vi "APE_tcp client.vi"(7 "Action":T1, 8 "error in":errorcluster, 9 "Command":string, 10 "TCP Port":u16=51019, 11 "Host":string) -> (0 "error out":errorcluster, 1 "Answer":string)   [LabVIEW 2026]
doc: "# #############################################################################\n# ATTENTION\n# #############################################################################\n#\n# This software is for guidance only. It is provided \"as is\".\n# It only aims at providing coding information to the customer in order for\n# them to save time. As a result no warranties, whether express, implied or\n# statutory, including, but not limited to implied warranties of\n# merchantability and fitness for a particular purpose apply to this software.\n# A·P·E Angewandte Physik und Elektronik GmbH shall not be held liable for any\n# direct, indirect or consequential damages with respect to any claims arising\n# from the content of such sourcecode and/or the use made by customers of the\n# coding information contained herein in connection with their products.\n#\n# File Version: 1.0\n#\n# Changelog:\n# 1.0 - Initial Version\n#\n# #############################################################################"
uses:
  APE codes/LabVIEW/LV13/Basic Example/cluster/tcp client action.ctl
  APE codes/LabVIEW/LV13/Basic Example/cluster/tcp client data cluster.ctl
  <vilib>/Utility/error.llb/Trim Whitespace One-Sided.vi
  <vilib>/regexp/Match Regular Expression.xnode
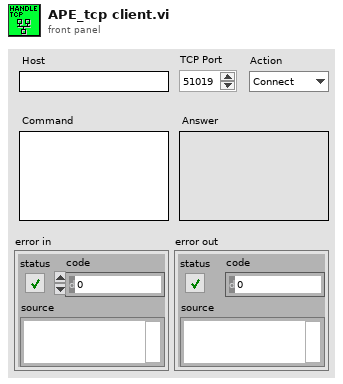
[diagram p1: front panel]
types:
  T1 = typedef "tcp client action.ctl" = enum16{"Connect", "Write", "Query", "Disconnect"}
  T2 = typedef "tcp client data cluster.ctl" = cluster{"connection ID":refnum<k5>, "Host":string, "TCP Port":u16}
  T3 = enum16{"Standard", "Buffered", "CRLF", "Immediate"}
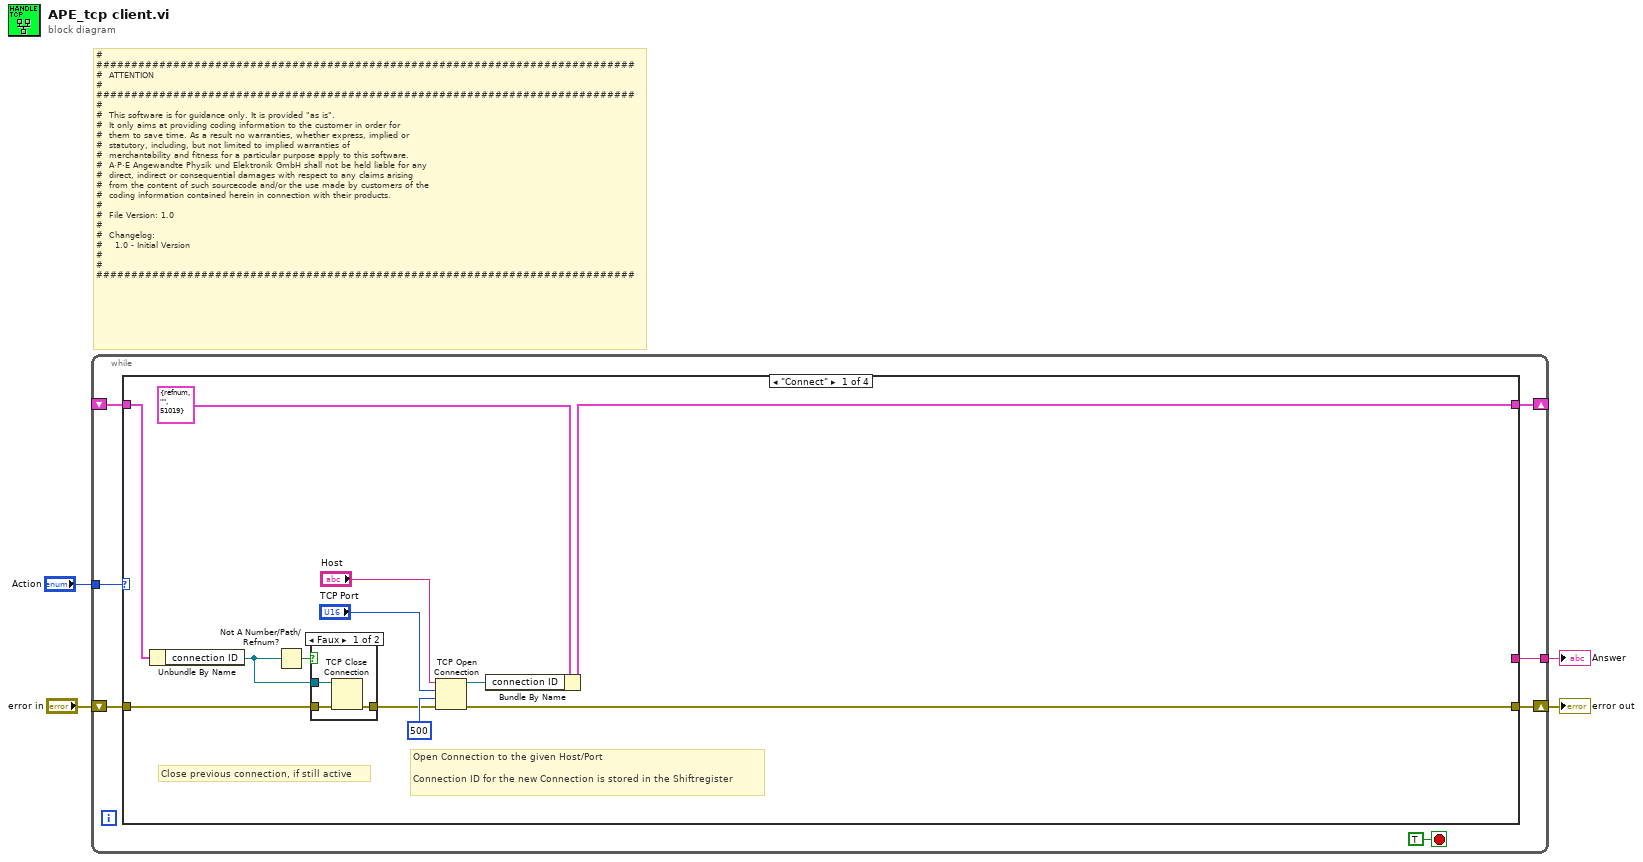
[diagram p0: block diagram]
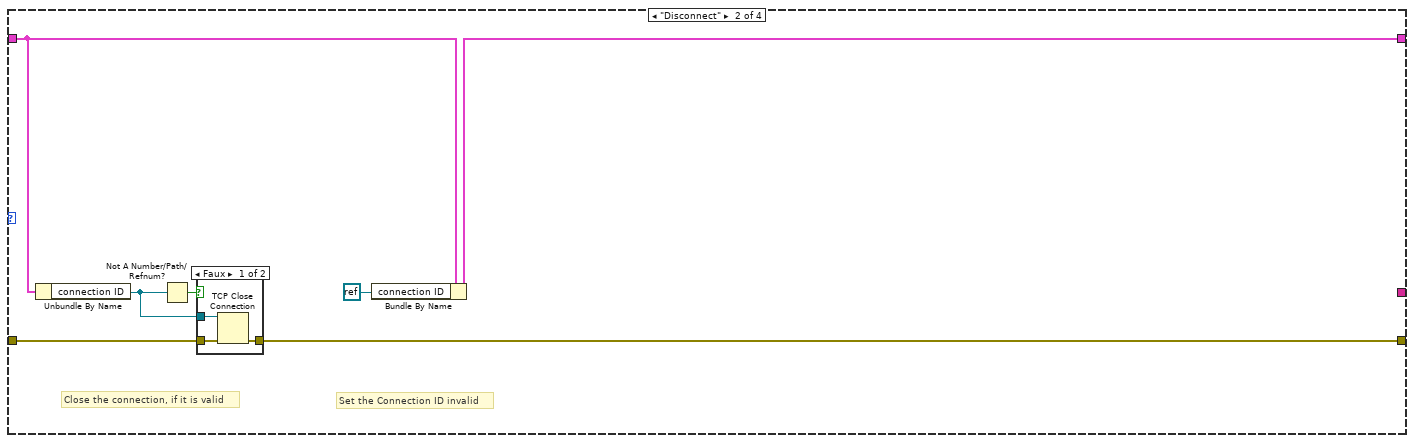
[diagram p3: hidden frame]
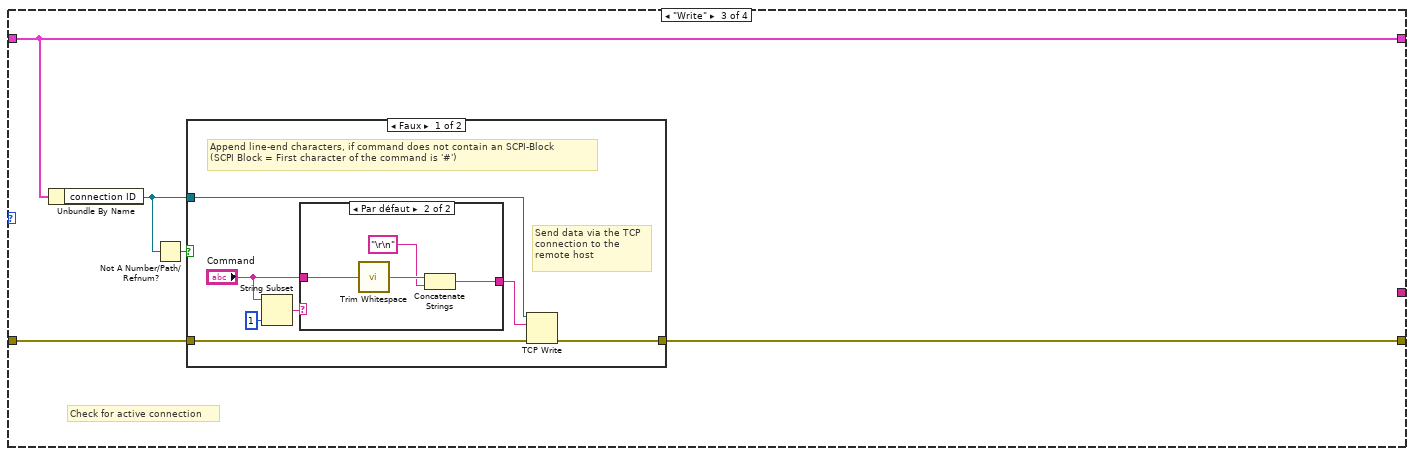
[diagram p5: hidden frame]
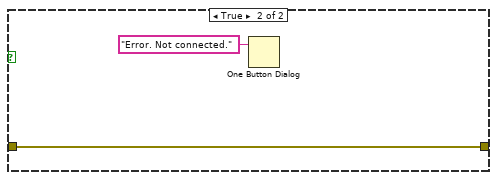
[diagram p7: hidden frame]
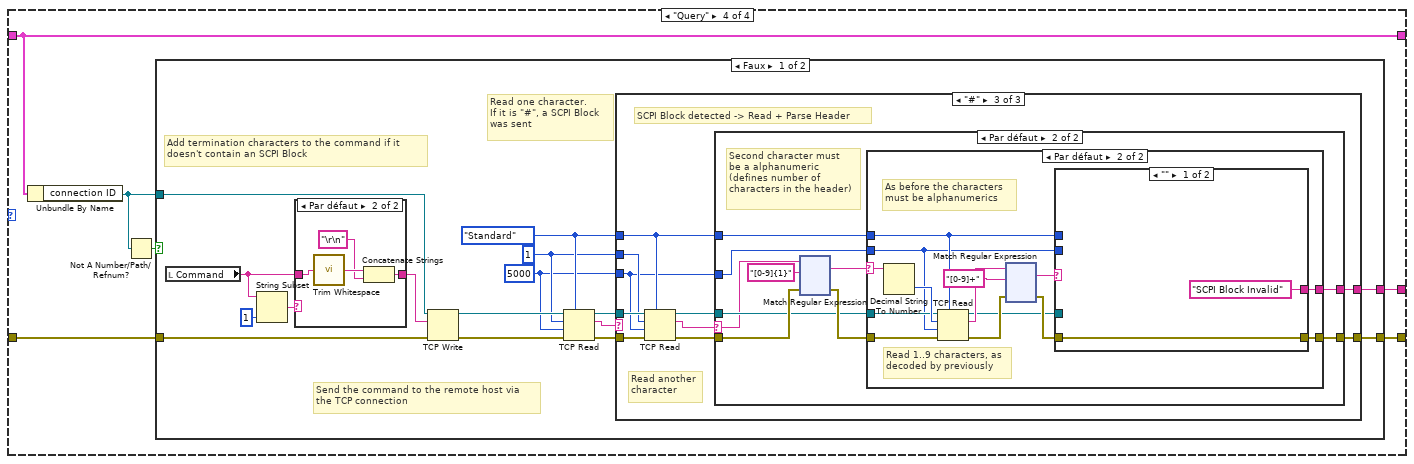
[diagram p8: hidden frame]
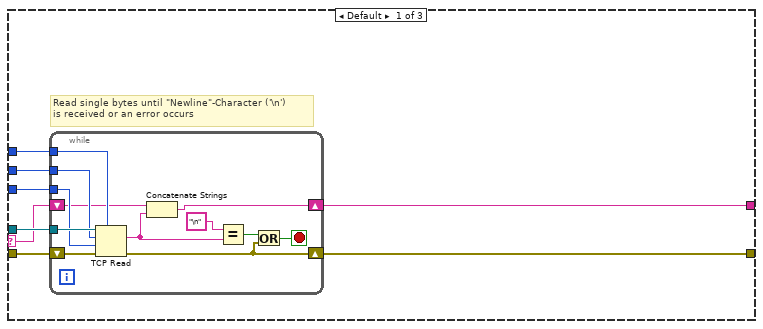
[diagram p9: hidden frame]
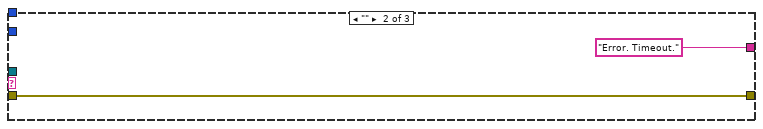
[diagram p10: hidden frame]
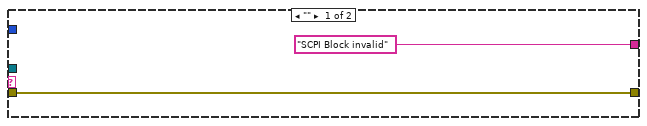
[diagram p11: hidden frame]
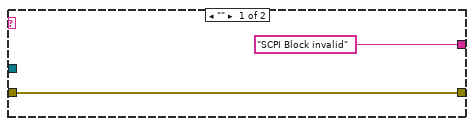
[diagram p12: hidden frame]
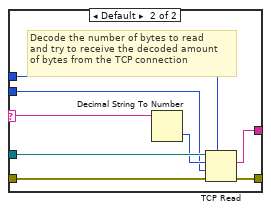
[diagram p13: hidden frame]
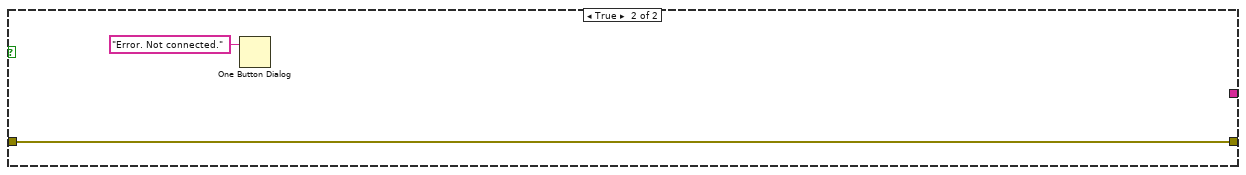
[diagram p15: hidden frame]
diagram:
  # "# #############################################################################\n#  ATTENTION\n# #############################################################################\n#\n#  This software is for guidance only. It is provided \"as is\".\n#  It only aims at providing coding information to the customer in order for\n#  them to save time. As a result no warranties, whether express, implied or\n#  statutory, including, but not limited to implied warranties of\n#  merchantability and fitness for a particular purpose apply to this software.\n#  A·P·E Angewandte Physik und Elektronik GmbH shall not be held liable for any\n#  direct, indirect or consequential damages with respect to any claims arising\n#  from the content of such sourcecode and/or the use made by customers of the\n#  coding information contained herein in connection with their products.\n#\n#  File Version: 1.0\n#\n#  Changelog:\n#    1.0 - Initial Version\n#\n# #############################################################################"
  n1 = while {
    shift-right: [w10] -> _
    shift-left: _ -> [w9]
    shift-right: [w8] -> w3
    shift-left: "error in" -> [w7]
    tunnel: "Action" -> [w6]
    tunnel: [w5] -> w1
    stop <- TRUE stop-if-true
    n2 = case shown="\"Connect\"" w6 {
      tunnel: [w15 w31 w40 w60] -> w10
      tunnel: w9 -> [w16 w28 w40 w60]
      tunnel: [w17 w30 w43 w63] -> w8
      tunnel: w7 -> [w20 w32 w42 w62]
      tunnel: [_ _ _ w58] -> w5
      frame "Connect" {
        # "Open Connection to the given Host/Port\n\nConnection ID for the new Connection is stored in the Shiftregister"
        # "Close previous connection, if still active"
        n3 = Unbundle By Name(w16) -> ("connection ID"=w21:refnum<k5>)
        n4 = Not A Number/Path/Refnum?(number/path/refnum=w21) -> (NaN/Path/Refnum?=w22:bool)
        n5 = case shown="Faux" w22 {
          tunnel: w21 -> [w26 _]
          tunnel: w20 -> [w25 w27]
          tunnel: [w24 w27] -> w18
          frame False {
            n6 = TCP Close Connection(connection ID=w26, error in (no error)=w25) -> (error out=w24:errorcluster)  [unwired: 1 in, 1 out]
          }
          frame True {
          }
        }
        n7 = TCP Open Connection(address="Host", remote port or service name="TCP Port", timeout ms (60000)=500, error in (no error)=w18) -> (connection ID=w14:refnum<k5>, error out=w17:errorcluster)  [unwired: 1 in]
        n8 = Bundle By Name(cluster=T2 {"connection ID"=refnum, "Host"="", "TCP Port"=51019}, "connection ID"=w14) -> (w15:T2)
      }
      frame "Disconnect" {
        # "Set the Connection ID invalid"
        # "Close the connection, if it is valid"
        n9 = Unbundle By Name(w28) -> ("connection ID"=w33:refnum<k5>)
        n10 = Not A Number/Path/Refnum?(number/path/refnum=w33) -> (NaN/Path/Refnum?=w34:bool)
        n11 = case shown="Faux" w34 {
          tunnel: w33 -> [w37 _]
          tunnel: w32 -> [w36 w38]
          tunnel: [w35 w38] -> w30
          frame False {
            n12 = TCP Close Connection(connection ID=w37, error in (no error)=w36) -> (error out=w35:errorcluster)  [unwired: 1 in, 1 out]
          }
          frame True {
          }
        }
        n13 = Bundle By Name(cluster=w28, "connection ID"=refnum<k0> refnum) -> (w31:T2)
      }
      frame "Write" {
        # "Check for active connection"
        n14 = Unbundle By Name(w40) -> ("connection ID"=w39:refnum<k5>)
        n15 = Not A Number/Path/Refnum?(number/path/refnum=w39) -> (NaN/Path/Refnum?=w41:bool)
        n16 = case shown="Faux" w41 {
          tunnel: [w46 w57] -> w43
          tunnel: w42 -> [w47 w57]
          tunnel: w39 -> [w45 _]
          frame False {
            # "Send data via the TCP\nconnection to the \nremote host"
            # "Append line-end characters, if command does not contain an SCPI-Block\n(SCPI Block = First character of the command is '#')"
            n17 = String Subset(string="Command", length (rest)=1 ("length (rest)")) -> (substring=w48:string)  [unwired: 1 in]
            n18 = case shown="Par défaut" w48 {
              tunnel: [w51 w55] -> w50
              tunnel: "Command" -> [w51 w54]
              frame "#" {
              }
              frame Default {
                n19 = call <vilib>:"Trim Whitespace.vi"("string"=w54) -> ("trimmed string"=w53:string)  [unwired: 1 in]
                n20 = Concatenate Strings(w53, "\r\n" ("termination")) -> (w55:string)
              }
            }
            n21 = TCP Write(connection ID=w45, data in=w50, error in (no error)=w47) -> (error out=w46:errorcluster)  [unwired: 1 in, 2 out]
          }
          frame True {
            n22 = One Button Dialog(message="Error. Not connected.") -> ()  [unwired: 1 in, 1 out]
          }
        }
      }
      frame "Query" {
        n23 = Unbundle By Name(w60) -> ("connection ID"=w59:refnum<k5>)
        n24 = Not A Number/Path/Refnum?(number/path/refnum=w59) -> (NaN/Path/Refnum?=w61:bool)
        n25 = case shown="Faux" w61 {
          tunnel: [w70 w390] -> w63
          tunnel: w62 -> [w76 w390]
          tunnel: w59 -> [w75 _]
          tunnel: [w64 _] -> w58
          frame False {
            w65 = 5000 ("timeout ms (25000)")
            w66 = 1 ("bytes to read")
            w67 = T3."Standard" ("mode (standard)")
            # "Send the command to the remote host via\nthe TCP connection"
            # "Add termination characters to the command if it \ndoesn't contain an SCPI Block"
            # "Read one character.\nIf it is \"#\", a SCPI Block \nwas sent"
            n26 = local read "Command"() -> (w74:string)
            n27 = String Subset(string=w74, length (rest)=1 ("length (rest)")) -> (substring=w77:string)  [unwired: 1 in]
            n28 = case shown="Par défaut" w77 {
              tunnel: [w384 w388] -> w79
              tunnel: w74 -> [w384 w387]
              frame "#" {
              }
              frame Default {
                n29 = call <vilib>:"Trim Whitespace.vi"("string"=w387) -> ("trimmed string"=w386:string)  [unwired: 1 in]
                n30 = Concatenate Strings(w386, "\r\n" ("termination")) -> (w388:string)
              }
            }
            n31 = TCP Write(connection ID=w75, data in=w79, error in (no error)=w76) -> (connection ID out=w72:refnum<k5>, error out=w73:errorcluster)  [unwired: 1 in, 1 out]
            n32 = TCP Read(connection ID=w72, bytes to read=w66, error in (no error)=w73, 7:w67, 9:w65) -> (connection ID out=w68:refnum<k5>, data out=w69:string, error out=w71:errorcluster)
            n33 = case shown="\"#\"" w69 {
              selector: w69 -> [w81 _ _]
              tunnel: w71 -> [w87 w100 w111]
              tunnel: [w86 w100 w106] -> w70
              tunnel: w68 -> [w85 _ w110]
              tunnel: w67 -> [w84 _ w103]
              tunnel: w66 -> [w83 _ w109]
              tunnel: w65 -> [w82 _ w102]
              tunnel: [w80 "Error. Timeout." ("data out") w105] -> w64
              frame Default {
                # "Read single bytes until \"Newline\"-Character ('\\n')\nis received or an error occurs"
                n34 = while {
                  tunnel: w85 -> [w98]
                  shift-right: [w88] -> w86
                  shift-left: w87 -> [w99]
                  tunnel: w84 -> [w97]
                  tunnel: w83 -> [w96]
                  tunnel: w82 -> [w95]
                  shift-right: [w93] -> w80
                  shift-left: w81 -> [w94]
                  stop <- w89 stop-if-true
                  n35 = TCP Read(connection ID=w98, bytes to read=w96, error in (no error)=w99, 7:w97, 9:w95) -> (data out=w92:string, error out=w88:errorcluster)  [unwired: 1 out]
                  n36 = Concatenate Strings(w94, w92) -> (w93:string)
                  n37 = Equal?(x="\n" ("y"), y=w92) -> (x = y?=w90:bool)
                  n38 = Or(x=w90, y=w88) -> (x .or. y?=w89:bool)
                }
              }
              frame "" {
              }
              frame "#" {
                # "Read another\ncharacter"
                # "SCPI Block detected -> Read + Parse Header"
                n39 = TCP Read(connection ID=w110, bytes to read=w109, error in (no error)=w111, 7:w103, 9:w102) -> (connection ID out=w104:refnum<k5>, data out=w107:string, error out=w108:errorcluster)
                n40 = case shown="Par défaut" w107 {
                  selector: w107 -> [_ w114]
                  tunnel: w108 -> [w112 w123]
                  tunnel: [w112 w116] -> w106
                  tunnel: ["SCPI Block invalid" w115] -> w105
                  tunnel: w104 -> [_ w120]
                  tunnel: w103 -> [_ w119]
                  tunnel: w102 -> [_ w118]
                  frame "" {
                  }
                  frame Default {
                    # "Second character must \nbe a alphanumeric\n(defines number of \ncharacters in the header)"
                    n41 = xnode "Match Regular Expression"("chaîne en entrée"=w114, "expression régulière"="[0-9]{1}" ("regular expression"), "entrée d'erreur"=w123) -> ("toute l'expression"=w117:string, "sortie d'erreur"=w121:errorcluster)  [unwired: 3 in, 3 out]
                    n42 = case shown="Par défaut" w117 {
                      selector: w117 -> [_ w136]
                      tunnel: w121 -> [w125 w138]
                      tunnel: w120 -> [_ w137]
                      tunnel: w119 -> [_ w128]
                      tunnel: w118 -> [_ w127]
                      tunnel: [w125 w131] -> w116
                      tunnel: ["SCPI Block invalid" ("data out") w126] -> w115
                      frame "" {
                      }
                      frame Default {
                        # "As before the characters \nmust be alphanumerics"
                        # "Read 1..9 characters, as \ndecoded by previously"
                        n43 = Decimal String To Number(string=w136) -> (number=w139:i32)  [unwired: 2 in, 1 out]
                        n44 = TCP Read(connection ID=w137, bytes to read=w139, error in (no error)=w138, 7:w128, 9:w127) -> (connection ID out=w129:refnum<k5>, data out=w133:string, error out=w134:errorcluster)
                        n45 = xnode "Match Regular Expression"("chaîne en entrée"=w133, "expression régulière"="[0-9]+" ("regular expression"), "entrée d'erreur"=w134) -> ("toute l'expression"=w130:string, "sortie d'erreur"=w132:errorcluster)  [unwired: 3 in, 3 out]
                        n46 = case shown="\"\"" w130 {
                          selector: w130 -> [_ w146]
                          tunnel: w132 -> [w140 w149]
                          tunnel: [w140 w148] -> w131
                          tunnel: w129 -> [_ w147]
                          tunnel: w128 -> [_ w145]
                          tunnel: w127 -> [_ w143]
                          tunnel: ["SCPI Block Invalid" ("data out") w142] -> w126
                          frame "" {
                          }
                          frame Default {
                            # "Decode the number of bytes to read\nand try to receive the decoded amount\nof bytes from the TCP connection"
                            n47 = Decimal String To Number(string=w146) -> (number=w144:i32)  [unwired: 2 in, 1 out]
                            n48 = TCP Read(connection ID=w147, bytes to read=w144, error in (no error)=w149, 7:w145, 9:w143) -> (data out=w142:string, error out=w148:errorcluster)  [unwired: 1 out]
                          }
                        }
                      }
                    }
                  }
                }
              }
            }
          }
          frame True {
            n49 = One Button Dialog(message="Error. Not connected.") -> ()  [unwired: 1 in, 1 out]
          }
        }
      }
    }
  }
  "error out" <- w3
  "Answer" <- w1
